vi "LVClass_Image data subtraction filtered image.vi"(0 "Image A":refnum<class "Image.lvclass">, 5 "ConfigFilePath":path, 11 "error in (no error)":errorcluster) -> (4 "Image out":refnum<class "Image.lvclass">, 15 "error out":errorcluster)   [LabVIEW 2020, in "Image.lvclass"]
doc: "Inplace subtraction : ImageA = ImageA \\- ImageB. Images must have the same\nsize, channels count and bits depth.\n\n--------------------------------------------------------------------------------\n\n<B>ImageAIn </B> : Image object.\n<B>ImageAOut </B> : Image object.\n<B>ImageB </B> : Image object.\n<B>ErrorIn </B> : Error\n<B>ErrorOut </B> : Error\n\n--------------------------------------------------------------------------------"
uses:
  Image.lvclass
  Image.lvclass/Image.ctl
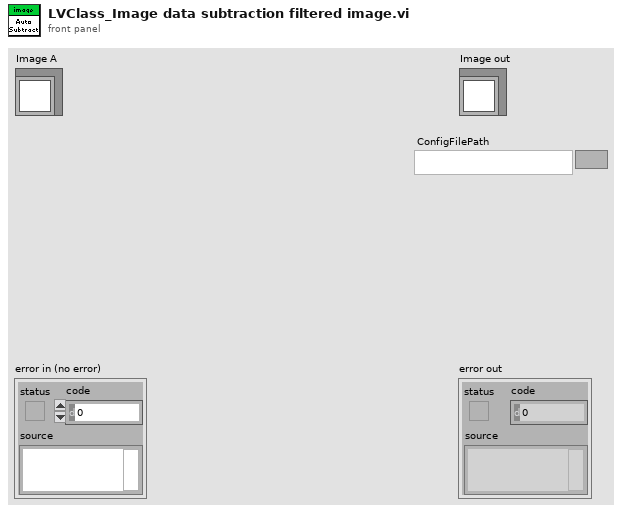
[diagram p1: front panel]
types:
  T1 = typedef "ClassID.ctl" = i64
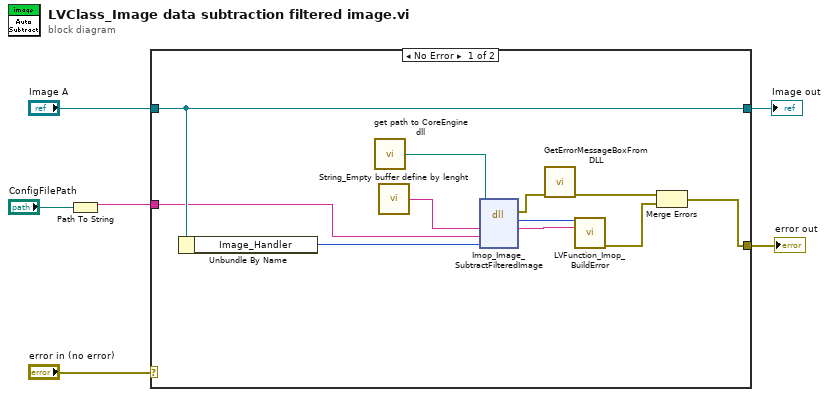
[diagram p0: block diagram]
diagram:
  n1 = Path To String(path="ConfigFilePath") -> (string=w1:string)
  n2 = case shown="No Error" "error in (no error)" {
    selector: "error in (no error)" -> [_ w19]
    tunnel: [w8 w19] -> w5
    tunnel: [w12 w18] -> w4
    tunnel: "Image A" -> [w12 w18]
    tunnel: w1 -> [w7 _]
    frame No Error {
      n3 = Unbundle By Name(w12) -> ("Image_Handler"=w11:T1)
      n4 = call "get path to CoreEngine dll.vi"() -> ("path to c_interface_vc100.dll"=w14:path)  [unwired: 12 in, 3 out]
      n5 = call "String_Empty buffer define by lenght.vi"() -> ("Empty buffer"=w17:string)  [unwired: 1 in]
      n6 = dll-call lib="D:/2_trunk/Soft_haso/ImOpCoreEngine4_LV2011/DLLs/ImopEngine4_vc100.dll" fn="Imop_Image_SubtractFilteredImage"(path in=w14, "message"=w17, "config_file_path"=w7, "Image"=w11) -> (error out=w13:errorcluster, "return type"=w16:i32, "message"=w15:string)  [unwired: 4 in, 1 out]
      n7 = call "GetErrorMessageBoxFromDLL.vi"("error IN"=w13) -> ("error OUT"=w10:errorcluster)  [unwired: 10 in]
      n8 = call "LVFunction_Imop_BuildError.vi"("code"=w16, "String to Prepend to source (\"\")"=w15) -> ("error out"=w9:errorcluster)  [unwired: 13 in]
      n9 = Merge Errors(w10, w9) -> (w8:errorcluster)
    }
    frame Error {
    }
  }
  "error out" <- w5
  "Image out" <- w4
